vi "New User (popup).vi"(8 "error in (no error)":errorcluster, 10 "User-data cluster":T1, 11 "file path (use dialog)":path) -> (0 "error out":errorcluster)   [LabVIEW 2012]
uses:
  SubVIs/typedef/User_Data_Cluster.ctl
  SubVIs/typedef/User Accounts.ctl
panel:
  out "Info Password not secure":bool
  out "Stop App?":bool
  in  "Cancel":bool
  in  "Usuario":string
  in  "Password":string
  in  "Reescriba la\nPassword":string
  in  "Admin":bool
  in  "Create":bool
  # "Log In attempt"
  # "of"
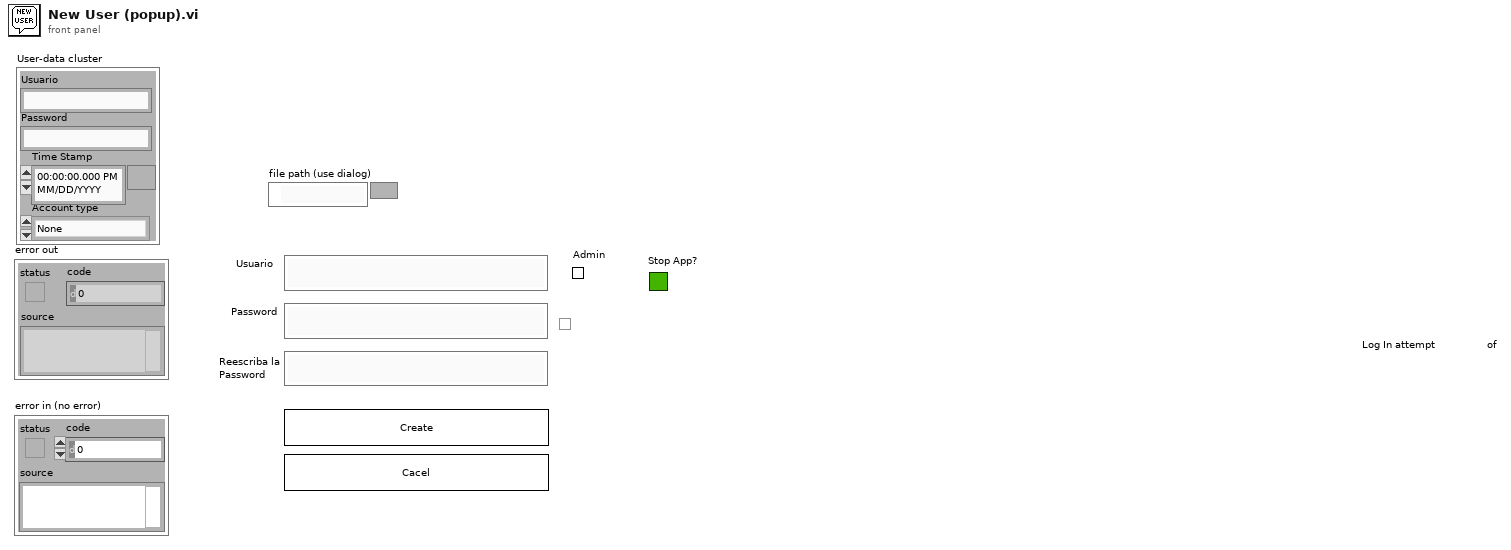
[diagram p1: front panel]
types:
  T1 = typedef "User_Data_Cluster.ctl" = cluster{"Usuario":string, "Password":string, "Account type":T2, "Time Stamp":timestamp}
  T2 = typedef "User Accounts.ctl" = enum16{"None", "User", "Admin"}
  T3 = cluster{"Usuario":string, "Password":string, "Account type":T2}
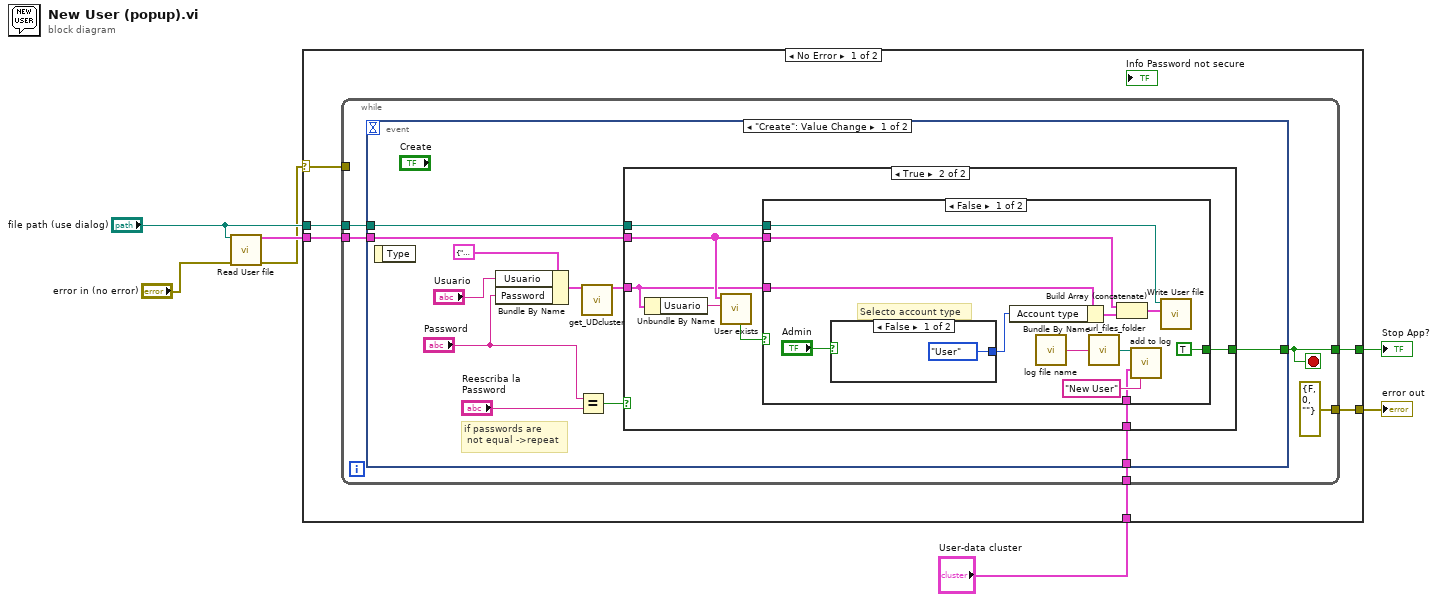
[diagram p0: block diagram]
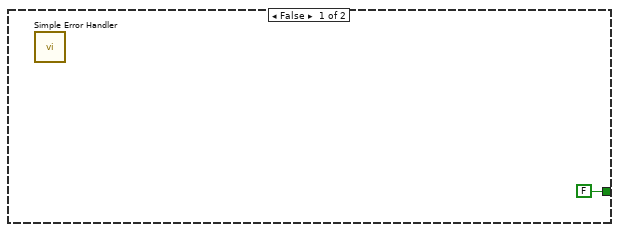
[diagram p2: hidden frame]
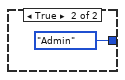
[diagram p3: hidden frame]
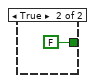
[diagram p4: hidden frame]
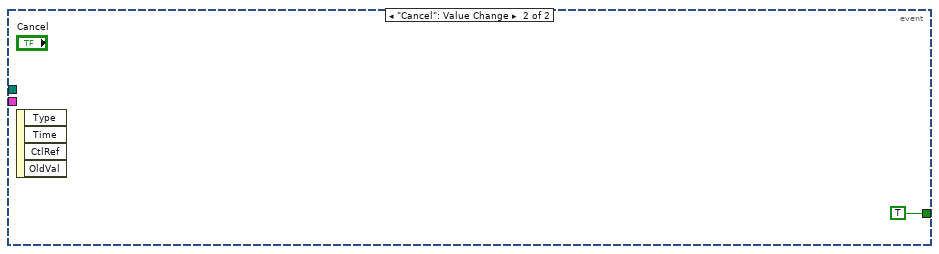
[diagram p5: hidden frame]
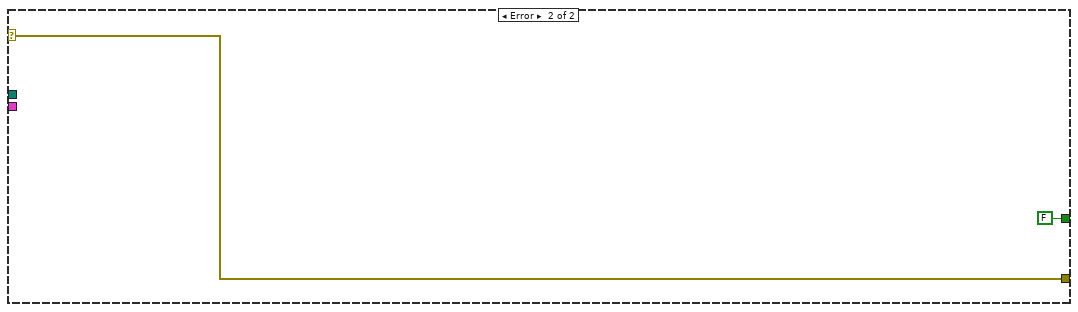
[diagram p6: hidden frame]
diagram:
  n1 = call "Read User file.vi"("file path (use dialog)"="file path (use dialog)", "error in"="error in (no error)") -> ("Array"=w5:T1[], "error out"=w3:errorcluster)  [unwired: 12 in]
  n2 = case shown="No Error" w3 {
    selector: w3 -> [w9 w55]
    tunnel: [w13 FALSE] -> w7
    tunnel: [w12 w55] -> w6
    tunnel: w5 -> [w11 _]
    tunnel: "file path (use dialog)" -> [w10 _]
    tunnel: "User-data cluster" -> [w8 _]
    frame No Error {
      n3 = while {
        tunnel: [w16] -> w13
        tunnel: w9 -> [_]
        tunnel: [errorcluster {"status"=FALSE, "code"=0, "source"=""} ("error in (no error)")] -> w12
        tunnel: w11 -> [w18]
        tunnel: w10 -> [w17]
        tunnel: w8 -> [w14]
        stop <- w16 stop-if-true
        n4 = event shown="[0] \"Create\": Value Change" {
          selector: _ -> [_ _]
          dyn-events: _ -> [_ _]
          timeout: _ -> [_ _]
          tunnel: w18 -> [w28 _]
          tunnel: w17 -> [w29 _]
          tunnel: [w22 TRUE] -> w16
          tunnel: w14 -> [w19 _]
          event "Create": Value Change {
            # "if passwords are\n not equal ->repeat"
            n5 = event-data() -> ()  [unwired: 1 in, 1 out]
            n6 = Bundle By Name(cluster=T3 {"Usuario"="", "Password"="", "Account type"=enum."None"} ("Data imput"), "Usuario"="Usuario", "Password"="Password") -> (w21:T3)
            n7 = Equal?(x="Password", y="Reescriba la\nPassword") -> (x = y?=w23:bool)
            n8 = call "get_UDcluster.vi"("Cluster"=w21) -> ("User-data cluster out"=w20:T1)  [unwired: 13 in, 1 out]
            n9 = case shown="True" w23 {
              tunnel: w29 -> [_ w37]
              tunnel: w28 -> [_ w35]
              tunnel: w20 -> [_ w34]
              tunnel: [FALSE w32] -> w22
              tunnel: w19 -> [_ w31]
              frame False {
                n10 = call <vilib>:"Simple Error Handler.vi"() -> ()  [unwired: 5 in, 5 out]
              }
              frame True {
                n11 = Unbundle By Name(w34) -> ("Usuario"=w36:string)
                n12 = call "User exists.vi"("user"=w36, "Array"=w35) -> ("exist?"=w33:bool)  [unwired: 6 in, 3 out]
                n13 = case shown="False" w33 {
                  tunnel: w37 -> [w47 _]
                  tunnel: w34 -> [w40 _]
                  tunnel: w35 -> [w45 _]
                  tunnel: [TRUE FALSE] -> w32
                  tunnel: w31 -> [w38 _]
                  frame False {
                    # "Selecto account type"
                    n14 = case shown="False" "Admin" {
                      tunnel: [User_Accounts."User" ("Account") User_Accounts."Admin" ("Account 2")] -> w48
                      frame False {
                      }
                      frame True {
                      }
                    }
                    n15 = Bundle By Name(cluster=w40, "Account type"=w48) -> (w44:T1)
                    n16 = call "log file name.vi"() -> ("file name"=w41:string)  [unwired: 15 in]
                    n17 = call "url_files_folder.vi"("file name"=w41) -> ("Path"=w42:path)  [unwired: 14 in]
                    n18 = Build Array (concatenate)(w45, w44) -> (w46:T1[])
                    n19 = call "add to log.vi"("Path"=w42, "User-data cluster"=w38, "Data"="New User" ("LogIn attempt")) -> ()  [unwired: 13 in]
                    n20 = call "Write User file.vi"("Array"=w46, "file path (use dialog)"=w47) -> ()  [unwired: 8 in, 2 out]
                  }
                  frame True {
                  }
                }
              }
            }
          }
          event "Cancel": Value Change {
            n21 = event-data() -> ()  [unwired: 1 in, 4 out]
          }
        }
      }
    }
    frame Error {
    }
  }
  "error out" <- w6
  "Stop App?" <- w7
